vi "cRIO_FPGA_COMMUNICATION Zähler_Zurücksetzen.vi"(3 "gewünschter Zälerwert":u16, 4 "Zähler":enum16{"Zähler 1", "Zähler 2", "Zähler 3"}(ring), 5 "Station Index":T1) -> (0 "Wert gesetzt":bool)   [LabVIEW 2013, in "cRIO_FPGA_COMMUNICATION.lvlib"]
uses:
  cRIO_FPGA_COMMUNICATION.lvlib
  TYPES/TYPE Station Index.ctl
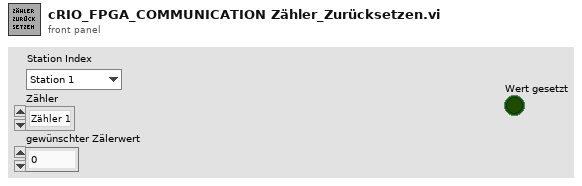
[diagram p1: front panel]
types:
  T1 = typedef "cRIO_FPGA_COMMUNICATION.lvlib/TYPE Station Index.ctl" = enum16{"Station 1", "Station 2", "Station 3", "Station 4", "Station 5", "Station 6", "Station 7", "Station 8", "Station 9", "Station 10", "Station 11", "Station 12", "Station 13", "Station 14", "Station 15", "Station 16", "Station 17", "Station 18", "Station 19", "Station 20"}
  T2 = enum16{"Init", "set Counter", "get Counter", "reset Counter", "configure Counter"}
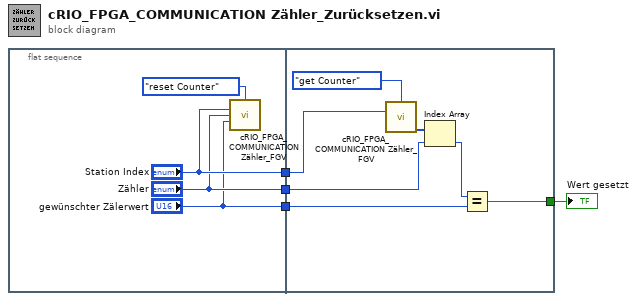
[diagram p0: block diagram]
diagram:
  n1 = flat-sequence {
    tunnel: ["Station Index"] -> w4
    tunnel: ["Zähler"] -> w3
    tunnel: ["gewünschter Zälerwert"] -> w2
    tunnel: w4 -> [w14]
    tunnel: w3 -> [w12]
    tunnel: w2 -> [w10]
    tunnel: [w9] -> w1
    frame #0 {
      n2 = call "cRIO_FPGA_COMMUNICATION Zähler_FGV.vi"("Set/Get/Configure"=T2."reset Counter", "Station Index"="Station Index", "Zähler"="Zähler", "gewünschter Zälerwert"="gewünschter Zälerwert") -> ()  [unwired: 10 in, 2 out]
    }
    frame #1 {
      n3 = call "cRIO_FPGA_COMMUNICATION Zähler_FGV.vi"("Set/Get/Configure"=T2."get Counter", "Station Index"=w14) -> ("Zählerwerte"=w13:u16[])  [unwired: 12 in, 1 out]
      n4 = Index Array(array=w13, index=w12) -> (element=w11:u16)
      n5 = Equal?(x=w11, y=w10) -> (x = y?=w9:bool)
    }
  }
  "Wert gesetzt" <- w1
